vi "removeEdge.vi"(0 "reference":refnum<class "SequenceDiagramGraph.lvclass">, 1 "edge":refnum<class "AbstractEdge.lvclass">, 5 "error in (no error)":errorcluster) -> (14 "reference out":refnum<class "SequenceDiagramGraph.lvclass">, 19 "error out":errorcluster)   [LabVIEW 2014, in "SequenceDiagramGraph.lvclass"]
uses:
  <resource>/Framework/Providers/Open_GDS/UML/SequenceDiagramGraph_class/SequenceDiagramGraph.lvclass
  <resource>/Framework/Providers/Open_GDS/UML/AbstractEdge_class/AbstractEdge.lvclass
  <resource>/Framework/Providers/Open_GDS/UML/Graph_class/Graph.lvclass
  <resource>/Framework/Providers/Open_GDS/UML/AbstractNode_class/AbstractNode.lvclass
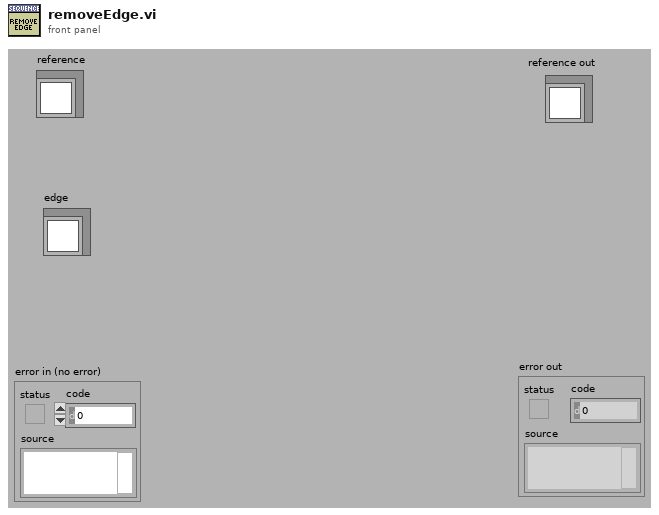
[diagram p1: front panel]
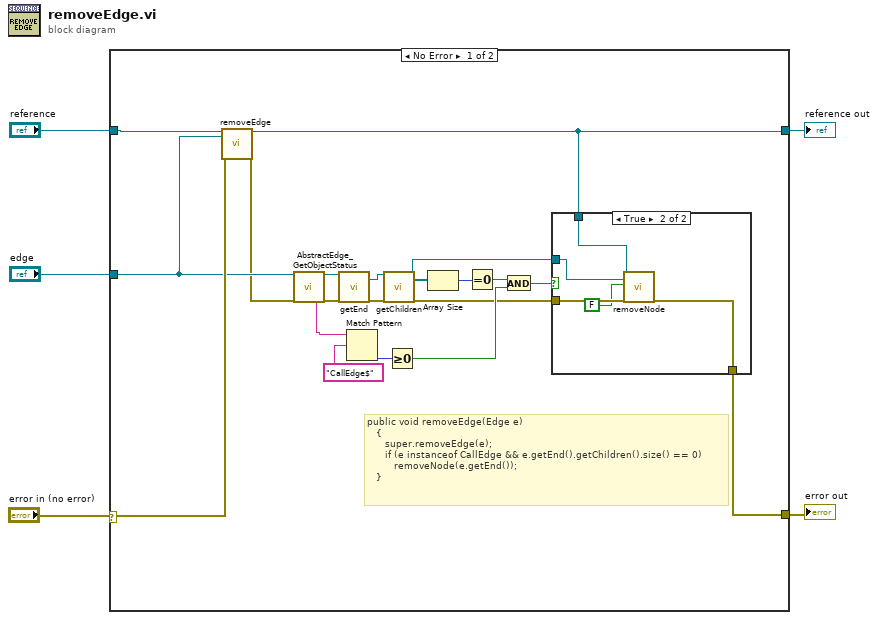
[diagram p0: block diagram]
diagram:
  n1 = case shown="No Error" "error in (no error)" {
    selector: "error in (no error)" -> [w10 w32]
    tunnel: "reference" -> [w11 w33]
    tunnel: [w25 w32] -> w4
    tunnel: [w7 w33] -> w3
    tunnel: "edge" -> [w9 _]
    frame No Error {
      # "public void removeEdge(Edge e)\n   {\n      super.removeEdge(e);\n      if (e instanceof CallEdge && e.getEnd().getChildren().size() == 0)\n         removeNode(e.getEnd());\n   }"
      n2 = call-parent "removeEdge.vi"("reference"=w11, "edge"=w9, "error in (no error)"=w10) -> ("reference out"=w7:refnum<class "SequenceDiagramGraph.lvclass">, "error out"=w8:errorcluster)  [unwired: 15 in]
      n3 = call <resource>:"AbstractEdge_GetObjectStatus.vi"("reference in"=w9, "error in (no error)"=w8) -> ("Class name"=w6:string, "reference out"=w23:refnum<class "AbstractEdge.lvclass">, "error out"=w22:errorcluster)  [unwired: 15 out]
      n4 = call-dynamic "getEnd.vi"("reference"=w23, "error in (no error)"=w22) -> ("endNode"=w21:refnum<class "AbstractNode.lvclass">, "error out"=w20:errorcluster)  [unwired: 14 in, 2 out]
      n5 = Match Pattern(string=w6, regular expression="CallEdge$") -> (offset past match=w16:i32)  [unwired: 4 out]
      n6 = call-dynamic "getChildren.vi"("reference"=w21, "error in (no error)"=w20) -> ("reference out"=w12:refnum<class "AbstractNode.lvclass">, "children"=w19:refnum<class "AbstractNode.lvclass">[], "error out"=w13:errorcluster)  [unwired: 14 in, 1 out]
      n7 = Greater Or Equal To 0?(x=w16) -> (x >= 0?=w15:bool)
      n8 = Array Size(array=w19) -> (size(s)=w18:i32)
      n9 = Equal To 0?(x=w18) -> (x = 0?=w17:bool)
      n10 = And(x=w17, y=w15) -> (x .and. y?=w14:bool)
      n11 = case shown="True" w14 {
        tunnel: w13 -> [w26 w31]
        tunnel: [w26 w29] -> w25
        tunnel: w12 -> [_ w30]
        tunnel: w7 -> [_ w28]
        frame False {
        }
        frame True {
          n12 = call-dynamic "removeNode.vi"("reference"=w28, "node"=w30, "RemoveChildrenIfAny(False)"=FALSE, "error in (no error)"=w31) -> ("error out"=w29:errorcluster)  [unwired: 14 in, 1 out]
        }
      }
    }
    frame Error {
    }
  }
  "reference out" <- w3
  "error out" <- w4
